vi "Obtain UI Message Queue.vi"(8 "error in (no error)":errorcluster, 11 "Name (unnamed)":string) -> (0 "error out":errorcluster, 3 "Message Queue":refnum<queue>)   [LabVIEW 2020, in "User Interface Utilities.lvlib" / "Message Queue.lvlib"]
doc: "Create a queue with the Message Cluster data type."
uses:
  Message Queue.lvlib
  Message.ctl
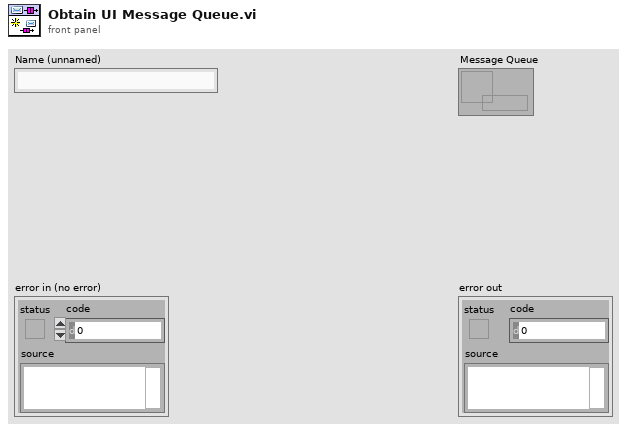
[diagram p1: front panel]
types:
  T1 = typedef "User Interface Utilities.lvlib/Message Queue.lvlib/Message.ctl" = cluster{"Action":string, "Data":variant}
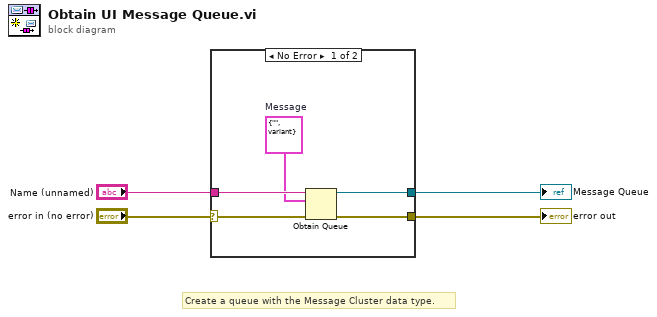
[diagram p0: block diagram]
diagram:
  # "Create a queue with the Message Cluster data type."
  n1 = case shown="No Error" "error in (no error)" {
    selector: "error in (no error)" -> [w6 w10]
    tunnel: [w9 _] -> w4
    tunnel: [w8 w10] -> w3
    tunnel: "Name (unnamed)" -> [w7 _]
    frame No Error {
      w5 = T1 {"Action"="", "Data"=variant}  # Message
      n2 = Obtain Queue(name (unnamed)=w7, element data type=w5, error in (no error)=w6) -> (queue out=w9:refnum<queue>, error out=w8:errorcluster)  [unwired: 2 in, 1 out]
    }
    frame Error {
    }
  }
  "Message Queue" <- w4
  "error out" <- w3
